vi "Balloon Fill Controller.vi"(8 "error in (no error)":errorcluster, 9 "Balloon Select":enum16{"Balloon 1", "Balloon 3", "Balloon 4"}(ring), 10 "Delay":u32, 11 "Queue in":refnum<queue>) -> ()   [LabVIEW 2020, in "CollectionSupport.lvlib"]
uses:
  CollectionSupport.lvlib
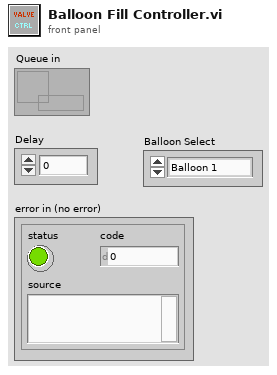
[diagram p1: front panel]
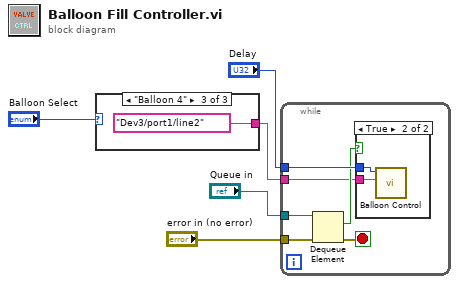
[diagram p0: block diagram]
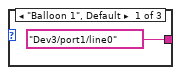
[diagram p2: hidden frame]
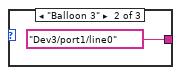
[diagram p3: hidden frame]
diagram:
  n1 = case shown="\"Balloon 4\"" "Balloon Select" {
    tunnel: [tag "Dev3/port1/line0" ("lines") tag "Dev3/port1/line0" ("lines") tag "Dev3/port1/line2" ("lines")] -> w2
    frame "Balloon 1", Default {
    }
    frame "Balloon 3" {
    }
    frame "Balloon 4" {
    }
  }
  n2 = while {
    tunnel: "Queue in" -> [w14]
    tunnel: "error in (no error)" -> [w13]
    tunnel: "Delay" -> [w11]
    tunnel: w2 -> [w9]
    stop <- w12 stop-if-true
    n3 = Dequeue Element(queue=w14, error in (no error)=w13) -> (element=w10:bool, error out=w12:errorcluster)  [unwired: 1 in, 2 out]
    n4 = case shown="True" w10 {
      tunnel: w11 -> [_ w16]
      tunnel: w9 -> [_ w15]
      frame False {
      }
      frame True {
        n5 = call "Balloon Control.vi"("lines"=w15, "Delay (ms)"=w16) -> ()  [unwired: 10 in]
      }
    }
  }
